vi "Mediana.vi"(0 "Datos_IN":dbl[][](array[numeric]), 5 "Error In":errorcluster) -> (14 "Min_Array":dbl[](array[numeric]), 19 "Error Out":errorcluster)   [LabVIEW 2013]
doc: "Finds the median value of the input sequence X by sorting the values of X and averaging the middle element(s) of the sorted array."
uses:
  <vilib>/Analysis/NI_AALBase.lvlib
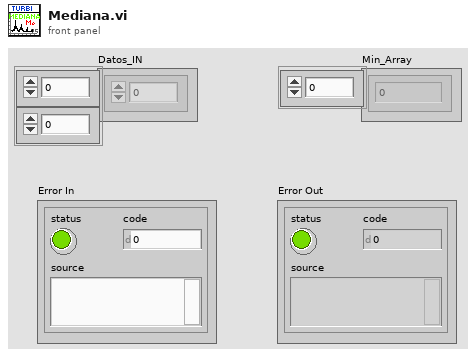
[diagram p1: front panel]
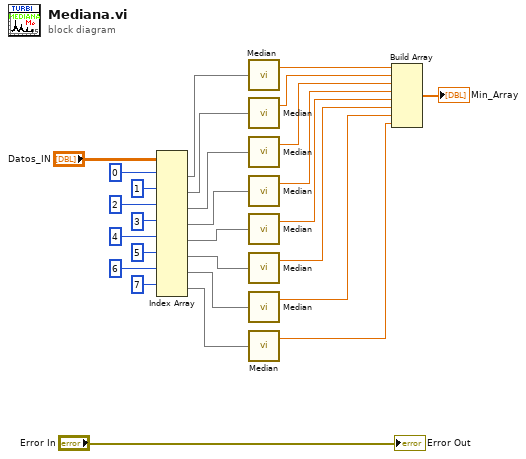
[diagram p0: block diagram]
diagram:
  n1 = Index Array(array="Datos_IN", index (row) #1=0 ("disabled index (col)"), index (row) #2=1 ("index (col)"), index (row) #3=2 ("index (col)"), index (row) #4=3 ("index (col)"), index (row) #5=4 ("index (col)"), index (row) #6=5 ("index (col)"), index (row) #7=6 ("index (col)"), index (row) #8=7 ("index (col)")) -> (element #1=w16:dbl[], element #2=w14:dbl[], element #3=w12:dbl[], element #4=w10:dbl[], element #5=w9:dbl[], element #6=w7:dbl[], element #7=w6:dbl[], element #8=w5:dbl[])  [unwired: 8 in]
  n2 = call <vilib>:"Median.vi"("X"=w16) -> ("median"=w15:dbl)  [unwired: 1 out]
  n3 = call <vilib>:"Median.vi"("X"=w14) -> ("median"=w13:dbl)  [unwired: 1 out]
  n4 = call <vilib>:"Median.vi"("X"=w12) -> ("median"=w11:dbl)  [unwired: 1 out]
  n5 = call <vilib>:"Median.vi"("X"=w10) -> ("median"=w8:dbl)  [unwired: 1 out]
  n6 = call <vilib>:"Median.vi"("X"=w9) -> ("median"=w4:dbl)  [unwired: 1 out]
  n7 = call <vilib>:"Median.vi"("X"=w7) -> ("median"=w3:dbl)  [unwired: 1 out]
  n8 = call <vilib>:"Median.vi"("X"=w6) -> ("median"=w2:dbl)  [unwired: 1 out]
  n9 = call <vilib>:"Median.vi"("X"=w5) -> ("median"=w1:dbl)  [unwired: 1 out]
  n10 = Build Array(w15, w13, w11, w8, w4, w3, w2, w1) -> (→"Min_Array":dbl[])
  "Error Out" <- "Error In"
